vi "Test Find Non Zero.vi"(8 "error in (no error)":errorcluster, 11 "Test Case In":refnum<class "Image.lvclass">) -> (0 "error out":errorcluster, 3 "Test Case Out":refnum<class "Image.lvclass">)   [LabVIEW 2020, in "g_ar_toolkit.test.lvlib" / "Image.lvclass"]
uses:
  Image.lvclass
  C:/Program Files (x86)/National Instruments/LabVIEW 2020/vi.lib/Astemes/LUnit/Test Case.lvclass
  g_ar_toolkit.common/Image Point (Integer).ctl
  <vilib>/Astemes/LUnit/Test Case.lvclass/Test Case.ctl
  4993e8ee-a06a-463a-9684-69129f64d5ce.vi
  <vilib>/Astemes/LUnit/Append Pass Result.vi
  <vilib>/Astemes/LUnit/Append Fail Result.vi
  <vilib>/Astemes/LUnit/Describe Comparison.vi
  4993e8ee-a06a-463a-9684-69129f64d5ce.vi/9c5d11cd-9439-4240-a1ee-d9baace9c924.vi
  <vilib>/Astemes/LUnit/Run In UI.vi
  <vilib>/Utility/error.llb/Clear Errors.vi
  g_ar_toolkit.common/Module Path.vi
  <vilib>/Utility/error.llb/Error Cluster From Error Code.vi
  <vilib>/Astemes/LUnit/Describe Variant.vi
  g_ar_toolkit.image/g_ar_toolkit.image.lvlib
  g_ar_toolkit.common/g_ar_toolkit.common.lvlib
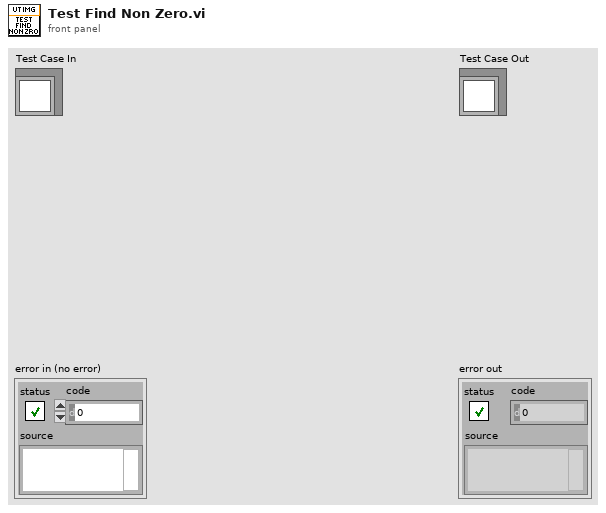
[diagram p1: front panel]
types:
  T1 = typedef "g_ar_toolkit.common.lvlib/Image Point (Integer).ctl" = cluster{"x":i32, "y":i32}
  T2 = typedef "g_ar_toolkit.image.lvlib/Greyscale Image.ctl" = refnum<data-value>
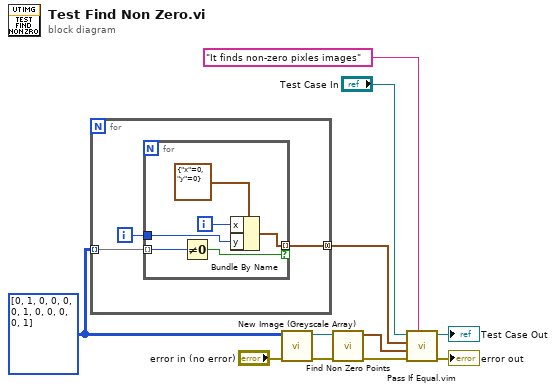
[diagram p0: block diagram]
diagram:
  w3 = u8[][] [[0, 1, 0, 0], [0, 0, 1, 0], [0, 0, 0, 1]] ("Greyscale Pixels (Default: Empty)")
  n1 = for {
    tunnel: w3 -> [w14] mode=indexing
    tunnel: [w12] -> w1 mode=concatenating
    i -> [w13]
    n2 = for {
      tunnel: w14 -> [w20] mode=indexing
      tunnel: w13 -> [w18]
      tunnel: [w17] -> w12 mode=indexing if=w16
      i -> [w19]
      n3 = Not Equal To 0?(x=w20) -> (x != 0?=w16:bool)
      n4 = Bundle By Name(cluster=T1 {"x"=0, "y"=0} ("Image Point"), "x"=w19, "y"=w18) -> (w17:T1)
    }
  }
  n5 = call "New Image (Greyscale Array).vi"("error in (no error)"="error in (no error)", "Greyscale Pixels (Default: Empty)"=w3) -> ("error out"=w5:errorcluster, "Greyscale Image"=w7:T2)  [unwired: 8 in]
  n6 = call "Find Non Zero Points.vi"("error in (no error)"=w5, "Greyscale Image-Source"=w7) -> ("error out"=w4:errorcluster, "Non Zero Points"=w2:T1[])  [unwired: 8 in]
  n7 = call "Pass If Equal.vim"("Description"="It finds non-zero pixles images", "error in (no error)"=w4, "Actual"=w2, "Expected"=w1, "LUnit Test Case In"="Test Case In") -> ("error out"=→"error out":errorcluster, "LUnit Test Case Out"=→"Test Case Out":refnum<class "Image.lvclass">)  [unwired: 5 in]
